vi "Write Display Mode.vi"(8 "error in (no error)":errorcluster, 9 "Display Mode":T1, 11 "Grove I2C LCD in":refnum<class "Grove I2C LCD.lvclass">) -> (0 "error out":errorcluster, 3 "Grove I2C LCD out":refnum<class "Grove I2C LCD.lvclass">)   [LabVIEW 2020, in "CTI-Peripheral.lvlib" / "Grove I2C LCD.lvclass"]
uses:
  Grove I2C LCD.lvclass
  HD44780 LCD/Display Mode.ctl
  Character LCD/Entry Shift.ctl
  Character LCD/Glyph Entry.ctl
  HD44780 LCD/Command.ctl
  Grove I2C LCD.lvclass/Grove I2C LCD.ctl
  HD44780 LCD/HD44780 LCD.lvlib
  Character LCD/Char LCD.lvclass
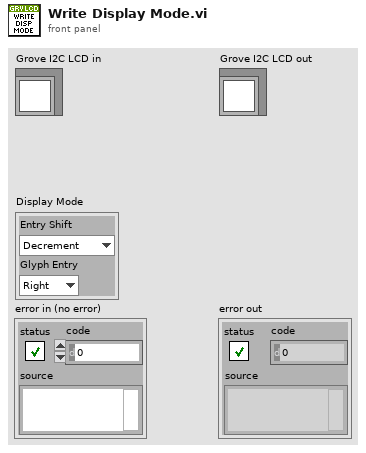
[diagram p1: front panel]
types:
  T1 = typedef "CTI-Peripheral.lvlib/HD44780 LCD.lvlib/Display Mode.ctl" = cluster{"Entry Shift":T2, "Glyph Entry":T3}
  T2 = typedef "CTI-Peripheral.lvlib/Char LCD.lvclass/Entry Shift.ctl" = enum8{"Decrement", "Increment"}
  T3 = typedef "CTI-Peripheral.lvlib/Char LCD.lvclass/Glyph Entry.ctl" = enum8{"Right", "Left"}
  T4 = typedef "CTI-Peripheral.lvlib/HD44780 LCD.lvlib/Command.ctl" = enum16{"ClearDisplay", "ReturnHome", "EntryModeSet", "DisplayControl", "CursorShift", "FunctionSet", "SetCGRamAddr", "SetDDRamAddr"}
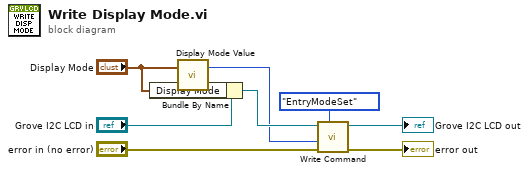
[diagram p0: block diagram]
diagram:
  n1 = Bundle By Name(cluster="Grove I2C LCD in", "Display Mode"="Display Mode") -> (w4:refnum<class "Grove I2C LCD.lvclass">)
  n2 = call "Display Mode Value.vi"("Display Mode"="Display Mode") -> ("DisplayMode"=w2:u8)  [unwired: 6 in]
  n3 = call "Write Command.vi"("Command"=Command."EntryModeSet", "error in (no error)"="error in (no error)", "Value"=w2, "Grove I2C LCD in"=w4) -> ("error out"=→"error out":errorcluster, "Grove I2C LCD out"=→"Grove I2C LCD out":refnum<class "Grove I2C LCD.lvclass">)  [unwired: 6 in]
